vi "Temperature Conversion.vi"(1 "Convert to C":bool, 2 "Temperature (F)":dbl) -> (0 "Numeric":dbl)   [LabVIEW 2020]
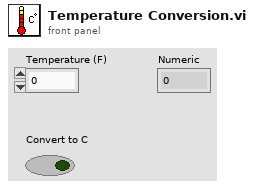
[diagram p1: front panel]
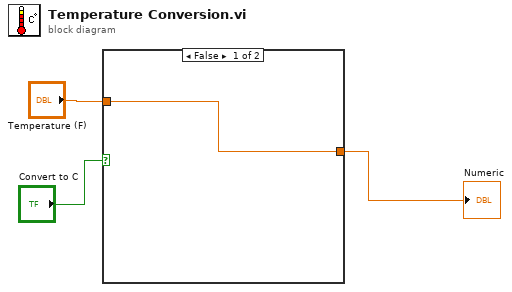
[diagram p0: block diagram]
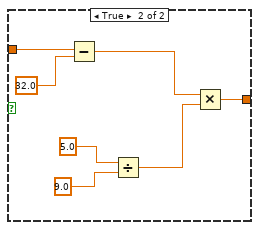
[diagram p2: hidden frame]
diagram:
  n1 = case shown="False" "Convert to C" {
    tunnel: [w4 w8] -> w3
    tunnel: "Temperature (F)" -> [w4 w5]
    frame False {
    }
    frame True {
      n2 = Subtract(x=w5, y=32.0) -> (x-y=w6:dbl)
      n3 = Divide(x=5.0, y=9.0) -> (x/y=w7:dbl)
      n4 = Multiply(x=w6, y=w7) -> (x*y=w8:dbl)
    }
  }
  "Numeric" <- w3
